vi "ReadEncoders(subvi).vi"(0 "Reset Encoders":bool, 5 "Cluster in":T1={FALSE, "Tick Count(uSec)"=0, "Counter Value"=[0, 0, 0, 0], "x-y"=[0, 0, 0, 0]}, 11 "error in (no error)":errorcluster) -> (2 "CM Oikea":dbl, 3 "CM Vasen":dbl, 4 "Tick Count(uSec)":u32 caption="Tick Count(Ticks)", 6 "CM Taka":dbl, 8 "output cluster":T2, 10 "CM Etu":dbl, 13 "Cluster Out":T1, 14 "Updated":bool, 15 "error out":errorcluster)   [LabVIEW 2018]
uses:
  <vilib>/myRIO/Common/Instrument Driver Framework/myRIO v1.0/Encoder/typedefs/Encoder Signal Mode.ctl
  <vilib>/myRIO/Instrument Drivers/Onboard IO/Encoder/typedefs/Encoder Reference.ctl
  <vilib>/myRIO/Common/Instrument Driver Framework/Utilities/typedefs/myRIO Generic Hardware Reference.ctl
  <vilib>/myRIO/Common/Instrument Driver Framework/Utilities/typedefs/Hardware Version Enum.ctl
  <vilib>/myRIO/Common/Instrument Driver Framework/Utilities/typedefs/myRIO v1.0 Reference.ctl
  <vilib>/myRIO/Common/Instrument Driver Framework/Utilities/typedefs/Generic FPGA Reference.ctl
  <vilib>/myRIO/Common/Instrument Driver Framework/myRIO v1.0/Encoder/typedefs/Encoder Channels Enum.ctl
  <vilib>/myRIO/Common/Instrument Driver Framework/myRIO v1.0/Encoder/typedefs/Encoder Configuration v1.0.ctl
  <vilib>/userdefined/High Color/nirio_resource_hc.ctl
  <vilib>/myRIO/Common/Instrument Driver Framework/Utilities/vis/Is FPGA Ref Available.vi
  <vilib>/myRIO/Common/Instrument Driver Framework/myRIO v1.0/Encoder/vis/myRIO v1.1 Open Encoder.vi
  <vilib>/myRIO/Instrument Drivers/Onboard IO/Encoder/vis/Read.vi
  <vilib>/myRIO/Common/Instrument Driver Framework/Utilities/vis/Validate Channels.vi
  <vilib>/myRIO/Common/Instrument Driver Framework/myRIO v1.0/Encoder/vis/myRIO v1.0 Reserve Encoder.vi
  <vilib>/myRIO/Common/Instrument Driver Framework/myRIO v1.0/Encoder/vis/myRIO v1.0 Build MUX Configuration Encoder.vi
  <vilib>/myRIO/Common/Instrument Driver Framework/myRIO v1.0/Resource Manager/vis/myRIO v1.0 Reserve Channel List.vi
  <vilib>/myRIO/Common/Instrument Driver Framework/myRIO v1.0/Resource Manager/vis/myRIO v1.0 Create Configuration List.vi
  <vilib>/myRIO/Common/Instrument Driver Framework/myRIO v1.0/Resource Manager/vis/myRIO v1.0 Reserve Channel.vi
  <vilib>/myRIO/Common/Instrument Driver Framework/myRIO v1.0/Resource Manager/vis/myRIO v1.0 Unreserve Channel.vi
  <vilib>/myRIO/Common/Instrument Driver Framework/myRIO v1.0/Resource Manager/vis/myRIO v1.0 Build Mutex Name.vi
  <vilib>/Utility/VariantDataType/GetNumericInfo.vi
  <vilib>/Utility/error.llb/Error Cluster From Error Code.vi
  <vilib>/myRIO/Common/Instrument Driver Framework/myRIO v1.0/myRIO v1.1 Open.vi
  <vilib>/myRIO/Common/Instrument Driver Framework/Utilities/vis/IO Manager.vi
  <vilib>/myRIO/Common/Instrument Driver Framework/Utilities/vis/Configuration Manager.vi
  <vilib>/myRIO/Common/Instrument Driver Framework/myRIO v1.0/Resource Manager/vis/myRIO v1.0 Configure IO.vi
  <vilib>/myRIO/Common/Instrument Driver Framework/myRIO v1.0/myRIO v1.0 Close.vi
  <vilib>/myRIO/Common/Instrument Driver Framework/myRIO v1.0/Encoder/vis/myRIO v1.0 Configure Encoder.vi
  <vilib>/myRIO/Common/Instrument Driver Framework/myRIO v1.0/Encoder/vis/myRIO v1.0 Read Encoder.vi
  <vilib>/myRIO/Express VI/Onboard IO/Encoder/Encoder Express VI.xnode
  <vilib>/myRIO/Instrument Drivers/Onboard IO/Encoder/vis/myRIO Encoder Open.xnode
  <vilib>/myRIO/Common/Instrument Driver Framework/myRIO v1.0/Encoder/typedefs/Encoder Count Direction Enum.ctl
  <vilib>/rvi/Arithmetic/AddSubMult/XNode/nirviSatArithmetic.xnode
  <vilib>/myRIO/Instrument Drivers/Onboard IO/Encoder/Encoder.lvlib
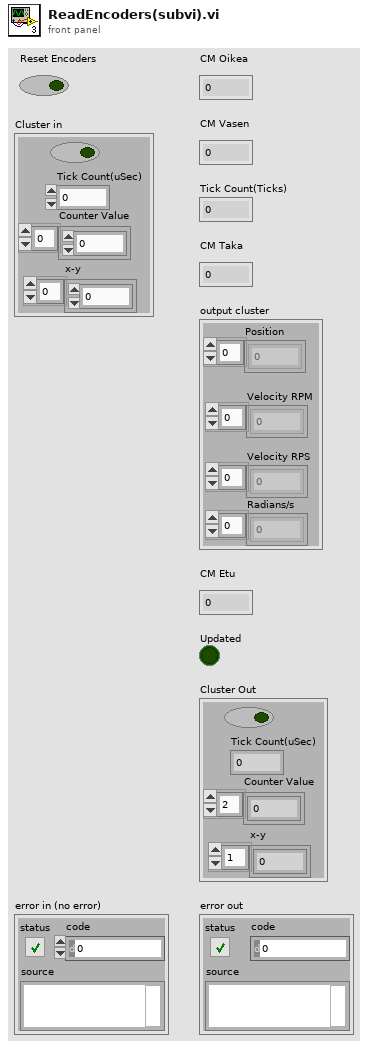
[diagram p1: front panel]
types:
  T1 = cluster{bool, "Tick Count(uSec)":u32, "Counter Value":i32[], "x-y":i32[]}
  T2 = cluster{"Position":i32[], "Velocity RPM":dbl[], "Velocity RPS":dbl[], "Radians/s":dbl[]}
  T3 = cluster{"Counter Value":i32[], dbl[], dbl[], dbl[]}
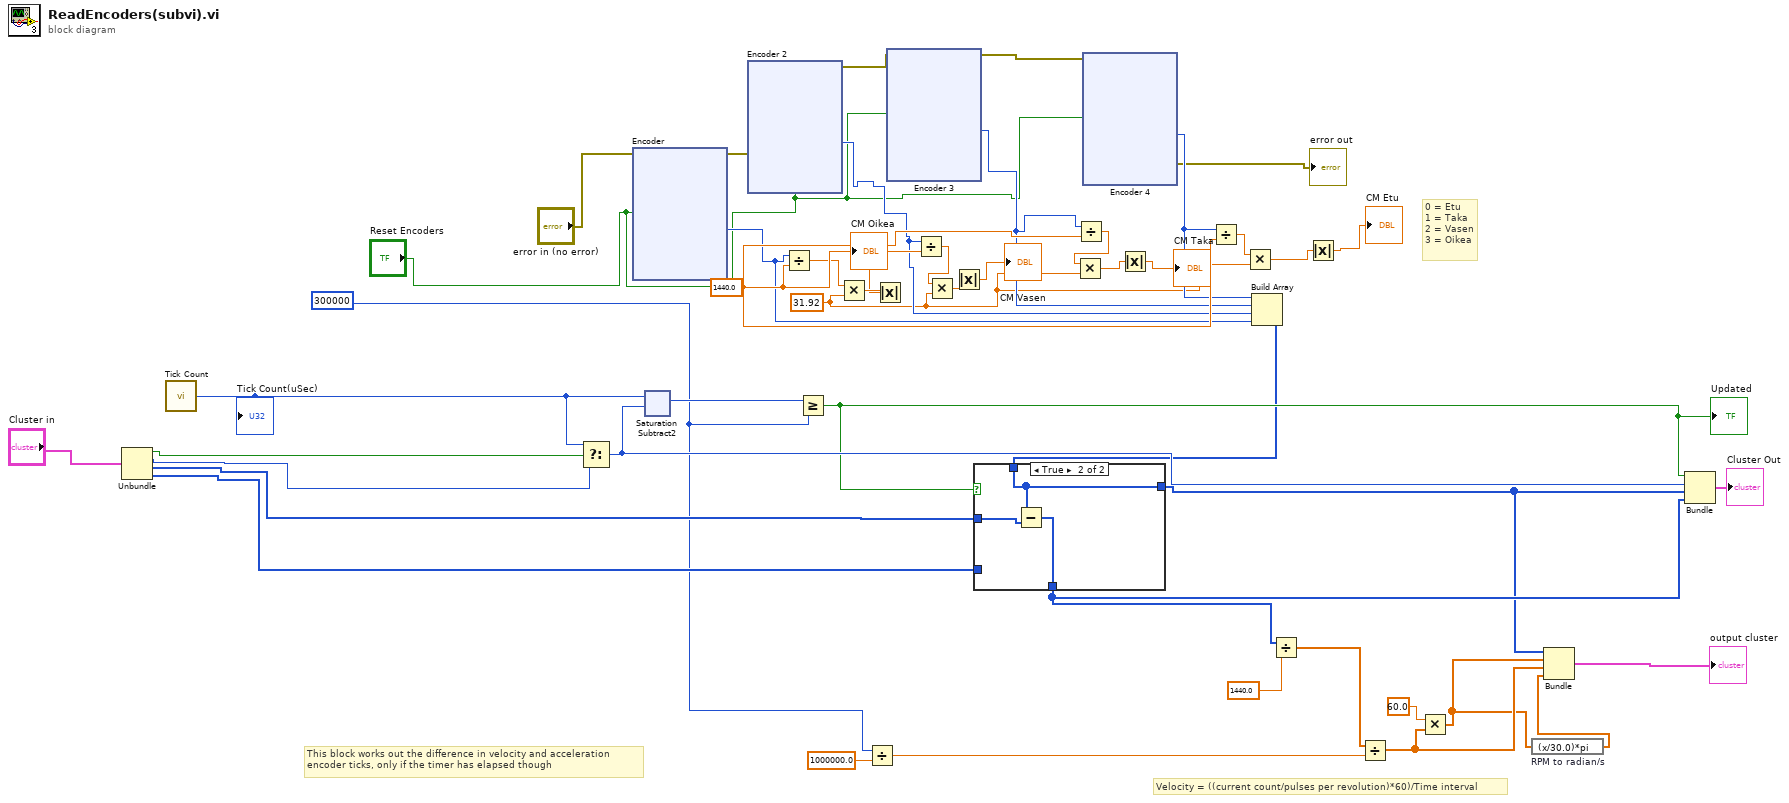
[diagram p0: block diagram]
diagram:
  w39 = 1440.0
  w32 = 31.92
  w2 = 300000
  # "0 = Etu\n1 = Taka\n2 = Vasen\n3 = Oikea"
  # "Velocity = ((current count/pulses per revolution)*60)/Time interval"
  # "This block works out the difference in velocity and acceleration \nencoder ticks, only if the timer has elapsed though"
  n1 = Unbundle("Cluster in") -> (w12:bool, "Tick Count(uSec)"=w11:u32, "Counter Value"=w10:i32[], "x-y"=w9:i32[])
  n2 = call "Tick Count"() -> ("Tick Count(uSec)"=w22:u32)
  "Tick Count(uSec)" <- w22
  n3 = Select(t=w22, s=w12, f=w11) -> (s? t:f=w21:u32)
  n4 = xnode "Encoder"("Reset Counter"="Reset Encoders", "error in (no error)"="error in (no error)") -> ("Counter Value"=w30:i32, "error out"=w16:errorcluster)  [unwired: 2 out]
  n5 = xnode ("Saturation Subtract2")("x"=w22, "y"=w21) -> ("x-y"=w17:u32)
  n6 = xnode "Encoder 2"("Reset Counter"="Reset Encoders", "error in (no error)"=w16) -> ("Counter Value"=w36:i32, "error out"=w5:errorcluster)  [unwired: 2 out]
  n7 = Divide(x=w30, y=w39) -> (x/y=w31:dbl)
  n8 = Greater Or Equal?(x=w17, y=w2) -> (x >= y?=w20:bool)
  "Updated" <- w20
  n9 = Multiply(x=w31, y=w32) -> (x*y=w41:dbl)
  n10 = Divide(x=w2, y=1000000.0) -> (x/y=w24:dbl)
  n11 = Absolute Value(x=w41) -> (abs(x)=→"CM Oikea":dbl)
  n12 = xnode "Encoder 3"("Reset Counter"="Reset Encoders", "error in (no error)"=w5) -> ("Counter Value"=w37:i32, "error out"=w4:errorcluster)  [unwired: 2 out]
  n13 = Divide(x=w36, y=w39) -> (x/y=w35:dbl)
  n14 = Multiply(x=w35, y=w32) -> (x*y=w42:dbl)
  n15 = Absolute Value(x=w42) -> (abs(x)=→"CM Vasen":dbl)
  n16 = Divide(x=w37, y=w39) -> (x/y=w34:dbl)
  n17 = Multiply(x=w34, y=w32) -> (x*y=w45:dbl)
  n18 = xnode "Encoder 4"("Reset Counter"="Reset Encoders", "error in (no error)"=w4) -> ("Counter Value"=w38:i32, "error out"=→"error out":errorcluster)  [unwired: 2 out]
  n19 = Absolute Value(x=w45) -> (abs(x)=→"CM Taka":dbl)
  n20 = Divide(x=w38, y=w39) -> (x/y=w33:dbl)
  n21 = Multiply(x=w33, y=w32) -> (x*y=w47:dbl)
  n22 = Build Array(w38, w37, w36, w30) -> (w15:i32[])
  n23 = case shown="True" w20 {
    tunnel: w10 -> [w48 w52]
    tunnel: [w49 w51] -> w25
    tunnel: w9 -> [w49 _]
    tunnel: [w48 w50] -> w23
    tunnel: w15 -> [_ w50]
    frame False {
    }
    frame True {
      n24 = Subtract(x=w50, y=w52) -> (x-y=w51:i32[])
    }
  }
  n25 = Divide(x=w25, y=1440.0) -> (x/y=w26:dbl[])
  n26 = Absolute Value(x=w47) -> (abs(x)=→"CM Etu":dbl)
  n27 = Divide(x=w26, y=w24) -> (x/y=w27:dbl[])
  n28 = Multiply(x=60.0 ("y"), y=w27) -> (x*y=w8:dbl[])
  n29 = expression code="(x/30.0)*pi" "RPM to radian/s"(w8) -> (w7:dbl[])
  n30 = Bundle("Counter Value"=w23, w8, w27, w7) -> (→"output cluster":T3)  [unwired: 1 in]
  n31 = Bundle(w20, "Tick Count(uSec)"=w21, "Counter Value"=w23, "x-y"=w25) -> (→"Cluster Out":T1)  [unwired: 1 in]
